vi "DIO's TestCode.vi"(8 "Step Text":string="String", 9 "Step Text":string="String", 11 "Step Text":string="String") -> (2 "DIO Output":string)   [LabVIEW 2014]
panel:
  out "DIO 3":bool
  out "DIO 2":bool
  out "DIO 1":bool
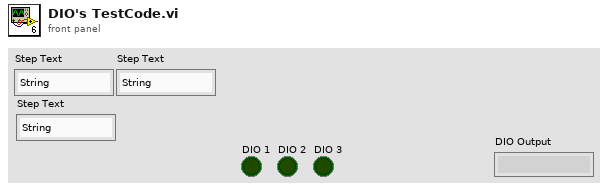
[diagram p1: front panel]
types:
  T1 = typedef "WPI_DigitalInputDevRef.ctl" = cluster{"DevStatus":errorcluster, "DIO Channel":T2, "Controller":T3}
  T2 = typedef "FPGA_DIOChannel.ctl" = enum8{"DIO 0", "DIO 1", "DIO 2", "DIO 3", "DIO 4", "DIO 5", "DIO 6", "DIO 7", "DIO 8", "DIO 9", "DIO MXP 0", "DIO MXP 1", "DIO MXP 2", "DIO MXP 3", "DIO MXP 4", "DIO MXP 5", "DIO MXP 6", "DIO MXP 7", "DIO MXP 8", "DIO MXP 9", "DIO MXP 10", "DIO MXP 11", "DIO MXP 12", "DIO MXP 13", "DIO MXP 14", "DIO MXP 15", "Invalid"}
  T3 = typedef "FPGA_TypedefDigitalModule.ctl" = enum16{"Controller 1"}
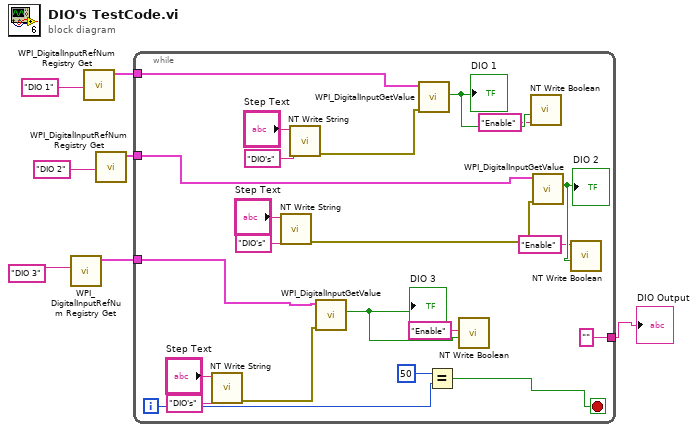
[diagram p0: block diagram]
diagram:
  n1 = call <vilib>:"WPI_DigitalInputRefNum Registry Get.vi"("refnum name"="DIO 3") -> ("DigitalInputDevRef"=w5:T1)  [unwired: 9 in, 1 out]
  n2 = call <vilib>:"WPI_DigitalInputRefNum Registry Get.vi"("refnum name"="DIO 1") -> ("DigitalInputDevRef"=w1:T1)  [unwired: 9 in, 1 out]
  n3 = call <vilib>:"WPI_DigitalInputRefNum Registry Get.vi"("refnum name"="DIO 2") -> ("DigitalInputDevRef"=w3:T1)  [unwired: 9 in, 1 out]
  n4 = while {
    tunnel: ["" ("DIO Output")] -> w7
    tunnel: w5 -> [w10]
    tunnel: w3 -> [w9]
    tunnel: w1 -> [w8]
    i -> [w13]
    stop <- w11 stop-if-true
    n5 = call <vilib>:"NT Write String.vi"("String"="DIO's", "Name"="Step Text") -> ("error out"=w23:errorcluster)  [unwired: 9 in]
    n6 = call <vilib>:"NT Write String.vi"("String"="DIO's", "Name"="Step Text") -> ("error out"=w26:errorcluster)  [unwired: 9 in]
    n7 = call <vilib>:"NT Write String.vi"("String"="DIO's", "Name"="Step Text") -> ("error out"=w29:errorcluster)  [unwired: 9 in]
    n8 = call <vilib>:"WPI_DigitalInputGetValue.vi"("error in (no error)"=w23, "DigitalInputDevRef"=w10) -> ("Value"=w15:bool)  [unwired: 7 in, 2 out]
    "DIO 3" <- w15
    n9 = call <vilib>:"WPI_DigitalInputGetValue.vi"("error in (no error)"=w29, "DigitalInputDevRef"=w8) -> ("Value"=w19:bool)  [unwired: 7 in, 2 out]
    "DIO 1" <- w19
    n10 = Equal?(x=50, y=w13) -> (x = y?=w11:bool)
    n11 = call <vilib>:"NT Write Boolean.vi"("Boolean"=w15, "Name"="Enable") -> ()  [unwired: 9 in, 1 out]
    n12 = call <vilib>:"NT Write Boolean.vi"("Boolean"=w19, "Name"="Enable") -> ()  [unwired: 9 in, 1 out]
    n13 = call <vilib>:"WPI_DigitalInputGetValue.vi"("error in (no error)"=w26, "DigitalInputDevRef"=w9) -> ("Value"=w17:bool)  [unwired: 7 in, 2 out]
    "DIO 2" <- w17
    n14 = call <vilib>:"NT Write Boolean.vi"("Boolean"=w17, "Name"="Enable") -> ()  [unwired: 9 in, 1 out]
  }
  "DIO Output" <- w7
